vi "worksheet set comments author lv.vi"(8 "error in (no error)":errorcluster, 10 "author":string, 11 "worksheet":u32) -> (0 "error out":errorcluster)   [LabVIEW 8.6]
doc: "void worksheet_set_comments_author_lv(lxw_worksheet worksheet, const char *author);"
uses:
  pending_lvxlsxwriter/xlsxwriter.dll
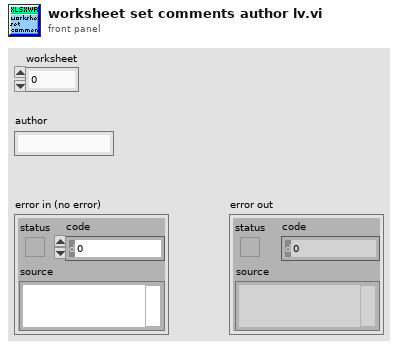
[diagram p1: front panel]
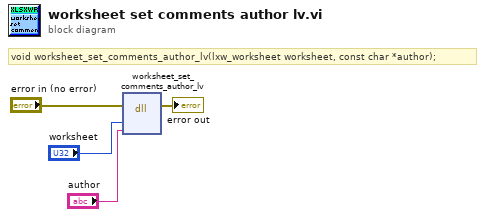
[diagram p0: block diagram]
diagram:
  # "void worksheet_set_comments_author_lv(lxw_worksheet worksheet, const char *author);"
  n1 = dll-call lib="C:/Users/WDAGUtilityAccount/Desktop/pending_lvxlsxwriter/xlsxwriter.*" fn="worksheet_set_comments_author_lv"(error in="error in (no error)", "worksheet"="worksheet", "author"="author") -> (error out=→"error out":errorcluster)  [unwired: 5 in, 1 out]
